vi "toString.vi"(8 "error in (no error)":errorcluster, 11 "Command in":refnum<class "Command.lvclass">) -> (0 "error out":errorcluster, 2 "String":string, 3 "Command out":refnum<class "Command.lvclass">)   [LabVIEW 2017, in "Message Interface.lvlib" / "Command.lvclass"]
uses:
  Command.lvclass
  Command.lvclass/Command.ctl
  iMessage/iMessage.lvclass
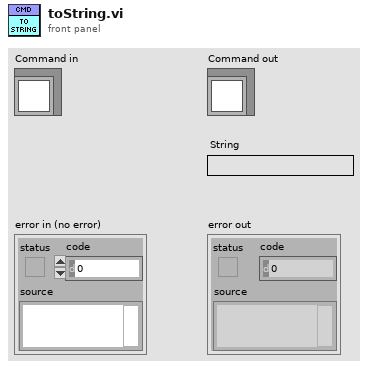
[diagram p1: front panel]
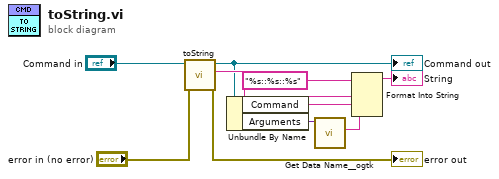
[diagram p0: block diagram]
diagram:
  n1 = call-parent "toString.vi"("error in (no error)"="error in (no error)", "iMessage in"="Command in") -> ("error out"=→"error out":errorcluster, "String"=w7:string, "iMessage out"=w4:refnum<class "Command.lvclass">)  [unwired: 7 in]
  "Command out" <- w4
  n2 = Unbundle By Name(w4) -> ("Command"=w3:string, "Arguments"=w1:variant)
  n3 = call <userlib>:"Get Data Name__ogtk.vi"("Data"=w1) -> ("Data Name"=w2:string)  [unwired: 8 in, 2 out]
  n4 = Format Into String(format string="%s::%s::%s", w7, w3, w2) -> (resulting string=→"String":string)  [unwired: 2 in, 1 out]
